vi "Global Fit Decays.vi"(6 "IRF":cluster{"t Array":dbl[], "IRF Array":dbl[]}, 8 "error in (no error)":errorcluster, 10 "Abort Fit":refnum<vi>, 11 "Decay Graph":refnum<vi>) -> (0 "Error Out":errorcluster, 1 "Reduced Chi^2":dbl, 2 "R^2":dbl, 3 "Best Fit Parameters":dbl[](array[numeric]), 4 "Fit Output Message":string, 5 "Aborted?":bool)   [LabVIEW 2021]
uses:
  AlliGator Settings List.ctl
  Fits/IRF(X)PSED/Decay Fit Options v2.ctl
  Fits/Decay Convolution/Decay Model.ctl
  Fits/Residual Type.ctl
  Fits/IRF(X)PSED/Fit Weights Type.ctl
  Fits/Non-linear Fitting Method v2.ctl
  Fits/Fit Calculation Method.ctl
  Fits/Non-linear Fitting Algorithm.ctl
  Fits/Global Fits/Global Fit Data.ctl
  Fits/Global Fits/Global Fit Parameters Information.ctl
  AlliGator Decay Fit Parameter Constraints 2.ctl
  Fits/IRF(X)PSED/Decay Fit Parameters In List.ctl
  AlliGator Variables List.ctl
  Graphs/XY Graph/XY Graph Add Multiplots with Names.vi
  Fits/Abort Fit Global.vi
  AlliGator Settings.lvlib
  Fits/Fits.lvlib
  AlliGator Decay Fit.lvlib
  Graphs/XY Graph/XY Graph Add-Ons.lvlib
  Time/Time.lvlib
  AlliGator Globals, Variables & Constants.lvlib
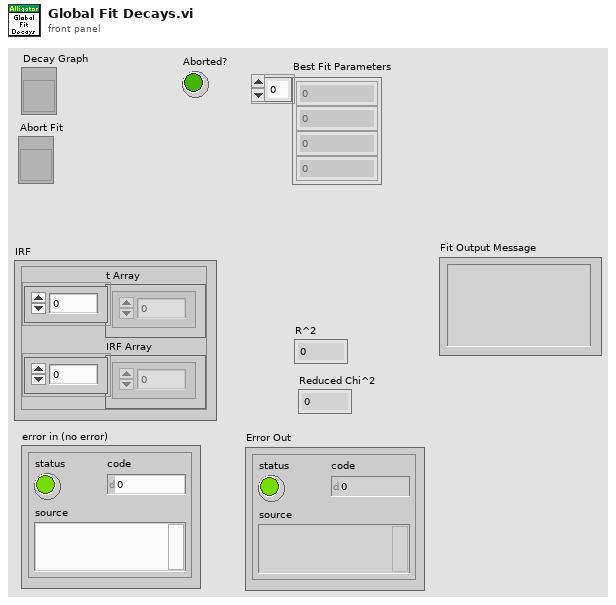
[diagram p1: front panel]
types:
  T1 = typedef "AlliGator Settings.lvlib/AlliGator Settings List.ctl" = enum16{"GUI:Visible Settings Tab", "GUI:Last Run Version", "Source Image:Use Image Histogram for Contrast", "Source Image:Low Count Pixels Rejection Options", "Source Image:High Count Pixels Rejection Options", "Source Image:Use Image Brightness", "Source Image:Blend Overlay with Image Background", "Source Image:Use Fixed ROI Diameter", "Source Image:ROI Diameter", "Source Image:ROI Center Color", "Source Image:Peak Threshold", "Source Image:Intensity Threshold", "Source Image:Image Binning Options", "Source Image:Image Smoothing Options", "Source Image:Image Histogram Active", "Source Image:Invert Binary Mask", "Source Image:Hot Pixel Removal", "Source Image:Overlay Analyzed ROI Center", "Source Image:Auto-Adjust Contrast", "Source Image:Histogram Lower Percentile", "Source Image:Histogram Upper Percentile", "Source Image:Save Source Image", "Source Image:Scale Bar Options", "Source Image:Image Resolution (Pixel Size)", "Source Image:Flatfield Correction", "Data Information:Gate Width", "Data Information:Nanotime Gate Separation", "Data Information:Macrotime Gate Separation", "Data Information:Gate Step", "Data Information:# Gates", "Data Information:Gate Image Exposure", "Data Information:Gate Image Integration", "Data Information:Gates to Skip", "Data Information:Gates to Keep", "Data Information:Define Gates to", "Data Information:Channel Name", "Data Information:Available Channel Names", "Data Information:Channel Arithmetic", "Data Information:Background File Subtraction", "Data Information:Background File", "Data Information:Background Scaling Factor", "Data Information:Background Pile-up Correction", "Data Information:Background Pixel Well Capacity", "Data Information:Laser Period", "Data Information:SYNC Period", "Data Information:Pile-up Correction", "Data Information:Pixel Well Capacity", "Data Information:Dataset Scaling Factor", "Fluorescence Decay_Decay Pre-Processing:Reverse Gates", "Fluorescence Decay_Decay Pre-Processing:Verbose Decay Pre-Processing", "Fluorescence Decay_Decay Pre-Processing:Use Decay Pre-Processing", "Fluorescence Decay_Decay Pre-Processing:Background Subtraction", "Fluorescence Decay_Decay Pre-Processing:Background Definition Range", "Fluorescence Decay_Decay Pre-Processing:Baseline Subtraction Method", "Fluorescence Decay_Decay Pre-Processing:Operations Order", "Fluorescence Decay_Decay Pre-Processing:Smoothing Parameter", "Fluorescence Decay_Decay Pre-Processing:Shift Decay", "Fluorescence Decay_Decay Pre-Processing:Decay Shift Parameters", "Fluorescence Decay_Decay Pre-Processing:Fold Decay", "Fluorescence Decay_Decay Pre-Processing:# Folds", "Fluorescence Decay_Decay Pre-Processing:1-Normalize Decay", "Fluorescence Decay_Decay Pre-Processing:[0-1]-Normalize Decay", "Fluorescence Decay_Decay Pre-Processing:Smoothen Decay", "Fluorescence Decay_Decay Pre-Processing:Extrapolate Decay", "Fluorescence Decay_Decay Pre-Processing:Use Periodicity", "Fluorescence Decay_Decay Pre-Processing:Use Cursors", "Fluorescence Decay_Decay Pre-Processing:Tail Fraction", "Fluorescence Decay_Decay Pre-Processing:Head Fraction", "Fluorescence Decay_Decay Pre-Processing:Additional Points", "Fluorescence Decay_Decay Pre-Processing:Straighten Decay", "Fluorescence Decay_Decay Pre-Processing:Constant Background", "Fluorescence Decay_Decay Pre-Processing:Pixel-Normalize Decay", "Fluorescence Decay_Advanced Analysis:Extract IRF instead of Decay", "Fluorescence Decay_Advanced Analysis:IRF Extraction Options", "Fluorescence Decay_Advanced Analysis:IRF Optimization Options", "Fluorescence Decay_Advanced Analysis:Square Pulse Options", "Fluorescence Decay_Advanced Analysis:IRF Order", "Fluorescence Decay_Advanced Analysis:IRF Time Constants", "Fluorescence Decay_Advanced Analysis:Wavelet Analysis Options", "Fluorescence Decay_Advanced Analysis:Average Lifetime Options", "Fluorescence Decay_Fit Options:Fit Options", "Fluorescence Decay_Fit Options:Use Legacy Fitting Approach", "Fluorescence Decay_Fit Options:Use Data Information Laser Period", "Fluorescence Decay_Fit Parameters:Displayed Fit Parameters", "Fluorescence Decay_Fit Parameters:Fit Parameter Constraints", "Fluorescence Decay_Fit Parameters:Export Tabulated Results", "Fluorescence Decay_Fit Parameters:MLE Baseline Offset Type", "Fluorescence Decay_Fit Parameters:MLE Baseline Offset", "Fluorescence Decay_Fit Parameters:Guess Parameter Names", "Fluorescence Decay_Fit Parameters:Guess Parameter Values", "Fluorescence Decay_Fit Parameters:Guess Parameters Options", "Fluorescence Decay_Styles:Show Last Decay Only", "Fluorescence Decay_Styles:Decay Graph Color Array", "Fluorescence Decay:Decay Graph Active", "Fluorescence Decay Statistics:Min Peak Value", "Fluorescence Decay Statistics:Reject Low Decay Peak Pixels", "Fluorescence Decay Statistics:Reject High Decay Peak Pixels", "Fluorescence Decay Statistics:Max Peak Value", "Time Traces:Use File Timestamp", "Time Traces:Time Step", "Time Traces:Use Intensity Correction File", "Time Traces:Intensity Correction File", "Phasor Plot:Phasor Plot Smoothing Options", "Phasor Plot:Phasor Plot Size", "Phasor Plot:Phasor Plot Graphics Options", "Phasor Plot:Cumulative Phasor Plot", "Phasor Plot:Use Phasor Brightness", "Phasor Plot:Blend Overlay with Phasor Background", "Phasor Plot:Save Phasor Plot", "Phasor Plot:Show References", "Phasor Plot:Phasor Ratio Decay Range", "Phasor Plot:Exponential Fading", "Phasor Plot:Phasor Ratio Reference Colors", "Phasor Plot:Reference Radius", "Phasor Plot:Show Color Map Vertices", "Phasor Plot:Phasor Plot Active", "Phasor Plot:Phasor Ratio Color Map Type", "Phasor Plot:Phasor Ratio Color Map", "Phasor Plot:Phasor Ratio Display Range", "Phasor Plot:Selected Image ROI(s)", "Phasor Plot:All Image ROIs", "Phasor Plot:Selected Phasor Plot ROI(s)", "Phasor Plot:All Phasor Plot ROIs", "Phasor Plot:Phasor Ratio Color-Coded Quantity", "Phasor Plot:Store Phasor Harmonics", "Phasor Plot:Draw Reference Segment", "Phasor Plot:User-Defined Quantity", "Phasor Graph:Phasor Frequency", "Phasor Graph:Phasor Ratio Type", "Phasor Graph:Pixel-level Phasor Computation", "Phasor Graph:Save Phasor Graph", "Phasor Graph:Phasor Graph Active", "Phasor Graph:Phasor SDV Options", "Phasor Calibration:Use Backup Calibration if needed", "Phasor Graph:Define Shortest Lifetime as", "Phasor Calibration:Backup Calibration Type", "Phasor Calibration:Calibration Type", "Phasor Calibration:Calibration Lifetime", "Phasor Calibration:Calibration Map Algorithm", "Single-Exponential Phasor Locus (SEPL):Gate Parameters", "Single-Exponential Phasor Locus (SEPL):User-defined Gate", "Single-Exponential Phasor Locus (SEPL):User-defined IRF", "Single-Exponential Phasor Locus (SEPL):Phasor Parameters", "Single-Exponential Phasor Locus (SEPL):Decay & IRF Parameters", "Single-Exponential Phasor Locus (SEPL):Display Parameters", "Lifetime Analysis:Decay Analysis Parameters", "Lifetime Analysis:Lifetime Map Active", "Plugins:Python Settings", "Miscellaneous:Verbose Mode", "Miscellaneous:Beep after Script", "Miscellaneous:Saved Image File Format", "Miscellaneous:Exported Gate Image Settings", "Miscellaneous:Include Loading in Timing", "Miscellaneous:Verbose Settings Mode", "Miscellaneous:Histogram Options", "Miscellaneous:Beep on Error", "Miscellaneous:# Logical Processors Used", "Miscellaneous:ROI Description Max Characters", "Miscellaneous:Verbose Error Mode", "Miscellaneous:Transparent Mask Color"}
  T2 = typedef "Fits.lvlib/Decay Fit Options v2.ctl" = cluster{"Show Fit Residuals":bool, "Fit Model":T3, "Residual Type":T4, "Max Decay Percentile":dbl, "Min Decay Percentile":dbl, "Show Full Decay":bool, "Weights":T5, "Fitting Method":T6, "Compute Parameter Uncertainties":bool, "Periodic Boundaries":bool, "Model Calculation":T7, "Period":dbl[unit], "Termination Criteria":cluster{"Max Iterations":i32, "Max Function Calls":i32, "Max Time":dbl[unit], "Function Tolerance":dbl, "Parameter Tolerance":dbl, "Gradient Tolerance":dbl, "Min Lambda":dbl, "Max Lambda":dbl, "Initial Tick Count":u32}, "Offset Resolution":dbl[unit], "Use Local IRF":bool, "Fitting Algorithm":T8}
  T3 = typedef "Fits.lvlib/Decay Model.ctl" = enum16{"1-Exponential", "2-Exponentials"}
  T4 = typedef "Fits.lvlib/Residual Type.ctl" = enum16{"Standard", "Normalized", "Reduced"}
  T5 = typedef "Fits.lvlib/Fit Weights Type.ctl" = enum16{"Unweighted", "1/Variance", "Best of All"}
  T6 = typedef "Fits.lvlib/Non-linear Fitting Method v2.ctl" = enum16{"Least Square", "Least Absolute Residual", "Bisquare", "MLE", "-", "Best of All"}
  T7 = typedef "Fits.lvlib/Fit Calculation Method.ctl" = enum16{"Simulation", "Convolution", "Integration"}
  T8 = typedef "Fits.lvlib/Non-linear Fitting Algorithm.ctl" = enum16{"Levenberg-Marquardt", "Trust-Region Dogleg"}
  T9 = cluster{"Max Iterations":i32, "Max Function Calls":i32, "Max Time":dbl[unit], "Function Tolerance":dbl, "Parameter Tolerance":dbl, "Gradient Tolerance":dbl, "Min Lambda":dbl, "Max Lambda":dbl, "Initial Tick Count":u32}
  T10 = typedef "XY Graph Add-Ons.lvlib/XY Graph Refnum.ctl" = refnum<vi>
  T11 = typedef "AlliGator Globals, Variables & Constants.lvlib/AlliGator Variables List.ctl" = enum16{"---- GUI ----", "Initialization Status", "State Indicators Refnum", "Original AlliGator Menu Items", "Current Action Loop State", "Script in progress", "Playback", "Loop Playback", "Search ROI Used", "Search ROI", "Decay Graph Max Legend Size", "Intensity Graph Max Legend Size", "Decay Statistics Graph Max Legend Size", "Phasor Graph Max Legend Size", "Phasor Ratio Graph Max Legend Size", "Lifetime Graph Max Legend Size", "---- Files ----", "Export Dataset Frames as Individual Files", "Show Batch Export Help Balloons", "Frames in Dataset", "ptu File Frame Start Indices", "Current Frame in Dataset", "Current Frame Timestamp", "------ Python Plugins ------", "Python Plugins Information", "Python Session", "Valid Python Session?", "---- Source Image ----", "Dataset Loaded", "Dataset Metadata", "Dataset Channel", "Dataset Data Description", "Background Dataset Metadata", "Background Dataset Channel", "Background Dataset Data Description", "Background File Subtraction", "Background File Path", "Background File Pile-up Correction", "Background File Pixel Well Capacity", "Background File Scaling Factor", "Source Image ROIs", "Current Source Image ROI", "Source Image ROI Event Refnum", "X_Source Image Display Range", "X_Source Image Palette Information", "Source Image Palette List", "Source Image Scale", "Current Dataset Load Settings", "Source Image:ROI Overlay Color", "---- Image Profile Window ----", "Image Profile:Overlay ROI in Source Image", "Image Profile Window Event Refnum", "Image Profile:IntensityType", "Image Profile:Intensity Average Type", "Image Profile:Intensity-weighted SDV", "Image Profile:Box Profile Type", "Image Profile Window Open", "Image Profile:Plotted Fit Parameter", "X_Type of Displayed Image", "X_Time Gate Slider", "Dataset Path", "Source Image Overlay to Erase", "Is Displayed Image Accumulated", "White Light Image Modified", "Mask Image Modified", "Macrotime Gate Separation", "------ Phasor Graph -------", "Phasor Graph:Show Line", "---- Phasor Plot ---", "Phasor Plot Parameters Changed", "FLI Dataset Modified since last Phasor Plot Calculation", "Phasor Harmonics Data", "Selected Phasor Harmonics", "Phasor Harmonic Manager Event Refnum", "Phasor Plot ROIs", "Current Phasor Plot ROI", "Phasor Plot ROI Event Refnum", "Phasor Plot Image Reference Points", "Phasor Plot Computed", "Phasor Plot Palette Information", "Phasor Plot Palette List", "Phasor Ratio Palette Information", "Phasor Ratio Palette List", "Phasor Image Scale", "Phasor Plot Image Overlay to Erase", "Phasor Plot Image Elements to Update", "Current Phasor Plot Calculation Parameters", "Current Phasor Calibration Options", "Reset Cumulated Phasor Plot", "Phasor Ratio Reference 1", "Phasor Ratio Lifetime Reference 1", "Phasor Ratio Reference 1 Frequency", "Phasor Ratio Reference 2", "Phasor Ratio Lifetime Reference 2", "Phasor Ratio Reference 2 Frequency", "---- Decay Analysis ----", "Number of Selected Decays to Fit", "LS Fit Results", "LAR Fit Results", "BS Fit Results", "Last Decay Max - Min", "Best Fit Parameters", "Best Fit Parameter Names", "Actual Size X", "Actual Size Y", "Binning X", "Binning Y", "Actual # Gates", "Dataset Number", "Gates to...", "Gates Skipped", "Gates to keep", "Gate Step", "Gate Separation", "Reversed Gates", "Pile-up Correction", "Pixel Well Capacity", "Background Subtracted", "Background Subtraction Method", "Background Definition Range", "Background File (deprecated)", "Number of Dataset Accumulated", "Array of Accumulated Dataset Paths", "Do Averaged Datasets", "Destination File Path", "Process Plot Target", "Use 1/D as Phasor Frequency", "---- Decay Fit Parameter Map -----", "Decay Fit Parameter Map Palette Information", "Decay Fit Parameter Map Palette List", "Local Decay Graph Window Event Refnum", "------- Local Decay Window ---------", "Use normalized IRF for convolution", "----- Miscellaneous ----", "Skippable Dialog Windows Status"}
  T12 = typedef "AlliGator Decay Analysis.lvlib/AlliGator Decay Fit.lvlib/AlliGator Decay Fit Parameter Constraints 2.ctl" = cluster{"Fit Parameter":T13, "Min Value":dbl, "Max Value":dbl, "Global":bool, "Used":bool}
  T13 = typedef "Fits.lvlib/Decay Fit Parameters In List.ctl" = enum16{"Offset", "Baseline", "A_1", "tau_1", "A_2", "tau_2"}
  T14 = typedef "Global Fit Data.ctl" = cluster{"Fit Data":variant, "Global Fit Parameter Information":T15, "# Points in Plots":i32[]}
  T15 = typedef "Fits.lvlib/Global Fit Parameters Information.ctl" = cluster{"Original Parameter Indices":i32[], "# Global Parameters":i32, "# Plot Specific Parameters":i32, "Global Parameter? Array":bool[]}
  T16 = cluster{"parameter minimum":dbl[], "parameter maximum":dbl[]}
  T17 = cluster{"t Array":dbl[], "Residual Array":dbl[]}[]
  T18 = typedef "Fits.lvlib/Non-linear Fit Output v3.ctl" = cluster{"best nonlinear fit":dbl[], "best fit parameters":dbl[], "R^2":dbl, "RMSE":dbl, "error out":errorcluster, "Fitting Method":T19, "number of function calls":i32, "number of iterations":i32, "covariance":T20, "Chi 2":dbl, "DOF":i32, "Fit Convergence Criterion":T21, "Fitting Algorithm":T8, "Weighted Fit":bool, "Gradient":dbl, "|Delta Chi 2|":dbl, "|Delta Chi 2|/Chi 2":dbl, "Max |Delta a| /|a|":dbl, "Lambda":dbl, "RSS":dbl, "AIC":dbl, "BIC":dbl, "Max number of function calls":i32, "Max number of iterations":i32, "IRF":T22, "IRF Normalization Factor":dbl, "Decay Normalization Factor":dbl}
  T19 = typedef "Fits.lvlib/Nonlinear Fit Method.ctl" = enum16{"Least Square", "Least Absolute Residual", "Bisquare", "MLE"}
  T20 = typedef "NI_Matrix.lvlib/RealMatrix.ctl" = dbl[][]
  T21 = typedef "Fits.lvlib/Convergence Criteria.ctl" = enum16{"Continue", "Tolerances Exceeded", "Max Time Exceeded", "Max Iterations Exceeded", "Max Function Evaluations Exceeded", "Scale Range Exceeded"}
  T22 = typedef "XY Graph Add-Ons.lvlib/XY Plot Data.ctl" = cluster{"X Array":dbl[], "Y Array":dbl[]}
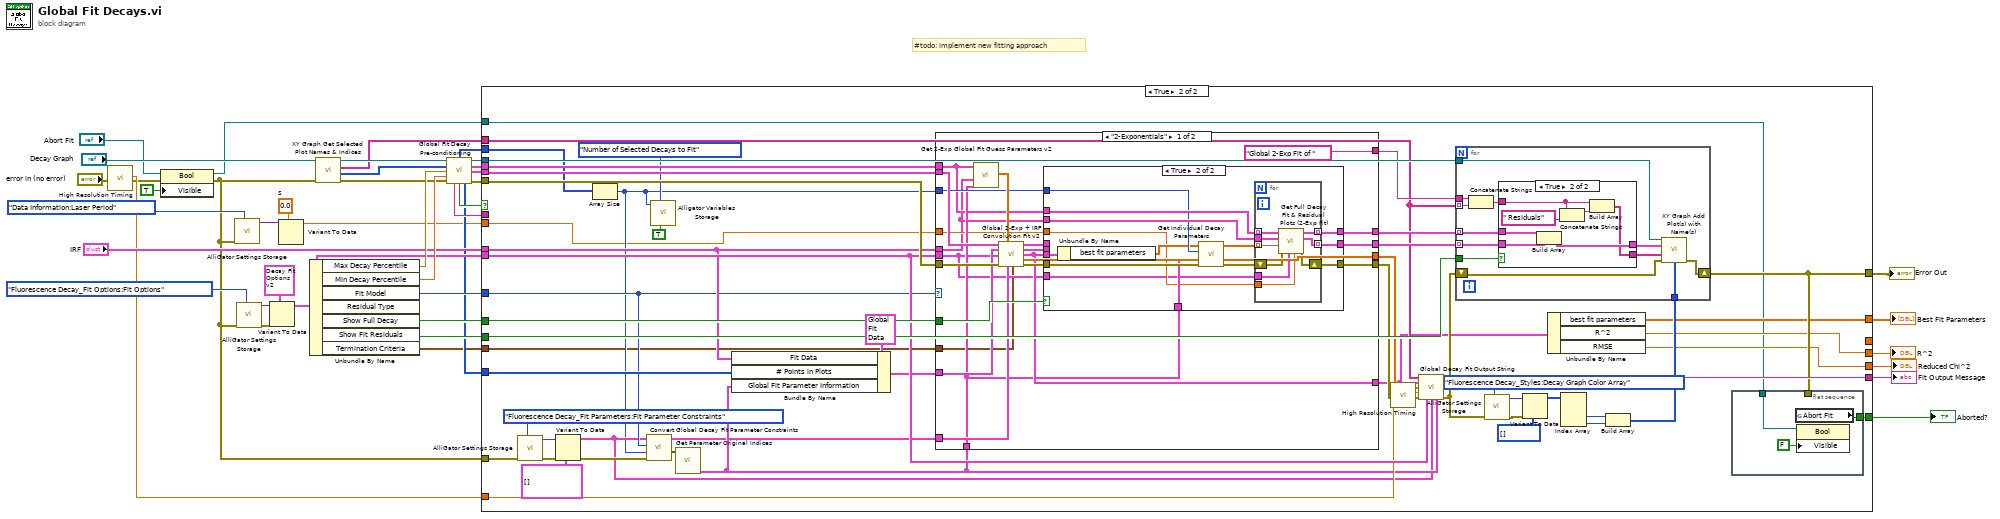
[diagram p0: block diagram]
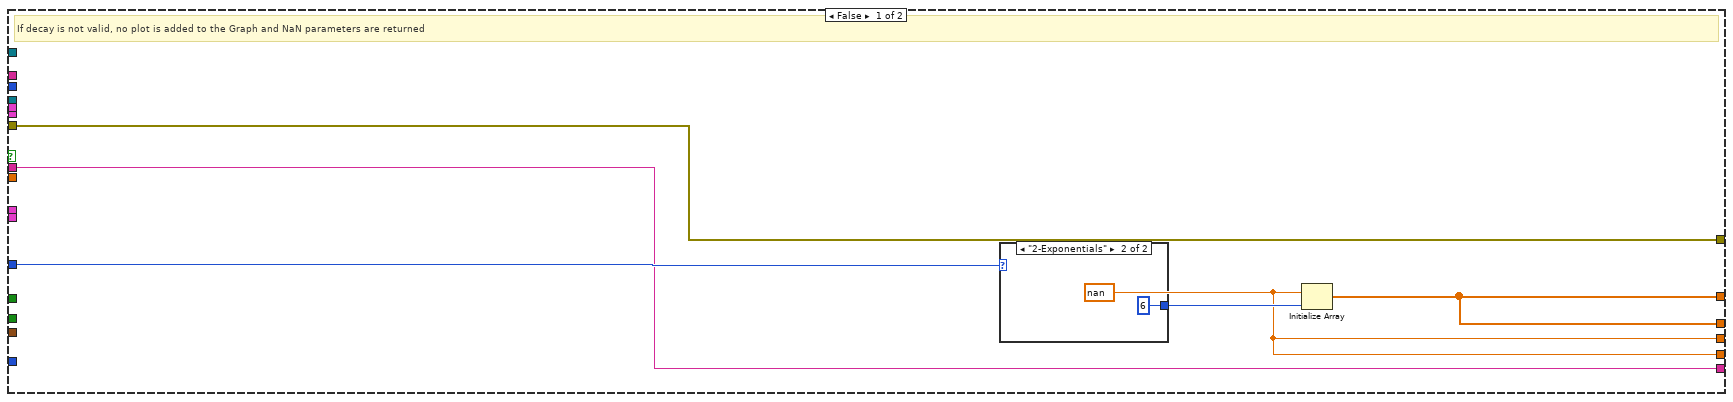
[diagram p2: hidden frame]
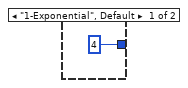
[diagram p3: hidden frame]
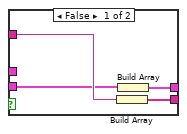
[diagram p4: hidden frame]
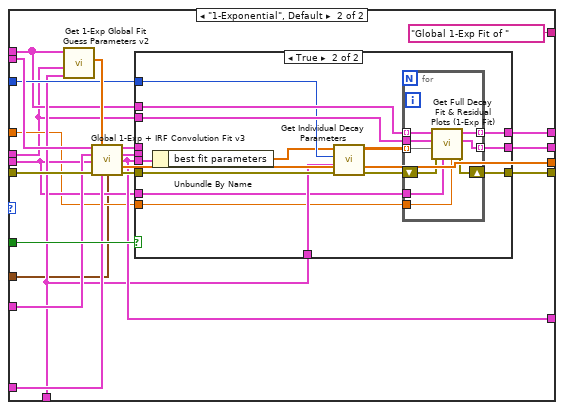
[diagram p6: hidden frame]
diagram:
  w8 = dbl[unit] 0.0  # s
  # "#todo: implement new fitting approach"
  n1 = call "High Resolution Timing.vi"("Error In"="error in (no error)") -> ("elapsed (relative) seconds"=w16:dbl, "Error Out"=w4:errorcluster)  [unwired: 16 in, 1 out]
  n2 = property class="Bool"(reference="Abort Fit", error in=w4, "Visible"=TRUE) -> (reference out=w2:refnum<vi>, error out=w3:errorcluster)
  n3 = call "AlliGator Settings Storage.vi"("AlliGator Settings List"=AlliGator_Settings_List."Data Information:Laser Period", "Error In"=w3) -> ("Variant Data out"=w9:variant)  [unwired: 8 in, 1 out]
  n4 = call "AlliGator Settings Storage.vi"("AlliGator Settings List"=AlliGator_Settings_List."Fluorescence Decay_Fit Options:Fit Options", "Error In"=w3) -> ("Error Out"=w37:errorcluster, "Variant Data out"=w38:variant)  [unwired: 8 in]
  n5 = Variant To Data(error in=w37, type=T2 {"Show Fit Residuals"=TRUE, "Fit Model"=enum."1-Exponential", "Residual Type"=enum."Standard", "Max Decay Percentile"=0.0, "Min Decay Percentile"=0.0, "Show Full Decay"=TRUE, "Weights"=enum."Unweighted", "Fitting Method"=enum."Least Square", "Compute Parameter Uncertainties"=TRUE, "Periodic Boundaries"=TRUE, "Model Calculation"=enum."Simulation", "Period"=1.2500000000000001e-08, "Termination Criteria"={"Max Iterations"=1000, "Max Function Calls"=0, "Max Time"=1000.0, "Function Tolerance"=1e-06, "Parameter Tolerance"=1e-06, "Gradient Tolerance"=0.0, "Min Lambda"=1e-06, "Max Lambda"=1e-06, "Initial Tick Count"=0}, "Offset Resolution"=1.2500000000000001e-08, "Use Local IRF"=TRUE, "Fitting Algorithm"=enum."Levenberg-Marquardt"} ("Fit Options"), Variant=w38) -> (data=w28:T2)  [unwired: 1 out]
  n6 = Variant To Data(type=w8, Variant=w9) -> (data=w7:dbl[unit])  [unwired: 1 in, 1 out]
  n7 = Unbundle By Name(w28) -> ("Max Decay Percentile"=w32:dbl, "Min Decay Percentile"=w31:dbl, "Fit Model"=w26:T3, "Show Full Decay"=w30:bool, "Show Fit Residuals"=w27:bool, "Termination Criteria"=w6:T9)  [unwired: 1 out]
  n8 = call "XY Graph Get Selected Plot Names & Indices.vi"("error in (no error)"=w3, "XYGraph in"="Decay Graph") -> ("error out"=w12:errorcluster, "Selected Plots"=w11:i32[], "Selected Plot Names"=w19:string[], "XYGraph out"=w24:T10)  [unwired: 5 in, 1 out]
  n9 = call "Global Fit Decay Pre-conditioning.vi"("XYGraph in"=w24, "Selected Plots"=w11, "Max Decay Percentile (1)"=w32, "Min Decay Percentile (0)"=w31, "error in (no error)"=w12) -> ("Index Max Array"=w20:i32[], "XYGraph out"=w42:refnum<vi>, "Full Decays"=w18:cluster{"t Array":dbl[], "Value Array":dbl[]}[], "Clipped Decays"=w22:cluster{"t Array":dbl[], "Value Array":dbl[]}[], "Message"=w23:string, "Is Valid?"=w29:bool, "# Points"=w13:i32[], "error out"=w14:errorcluster)  [unwired: 1 in, 2 out]
  n10 = case shown="True" w29 {
    tunnel: w42 -> [_ w103]
    tunnel: [w48 w85] -> w41
    tunnel: [w43 w100] -> w40
    tunnel: [w45 w56] -> w35
    tunnel: [w45 _] -> _
    tunnel: [w44 w55] -> w34
    tunnel: w26 -> [w47 w79]
    tunnel: [w44 w54] -> w33
    tunnel: "IRF" -> [_ w83]
    tunnel: w30 -> [_ w96]
    tunnel: w27 -> [_ w104]
    tunnel: w14 -> [w48 w95]
    tunnel: w28 -> [_ w93]
    tunnel: w23 -> [w43 _]
    tunnel: w22 -> [_ w92]
    tunnel: w20 -> [_ w59]
    tunnel: w19 -> [_ w90]
    tunnel: w18 -> [_ w91]
    tunnel: w16 -> [_ w88]
    tunnel: [_ w86] -> w15
    tunnel: w13 -> [_ w82]
    tunnel: w3 -> [_ w73]
    tunnel: w7 -> [_ w53]
    tunnel: w6 -> [_ w52]
    tunnel: w2 -> [_ w51]
    frame False {
      w44 = nan ("element")
      # "If decay is not valid, no plot is added to the Graph and NaN parameters are returned"
      n11 = case shown="\"2-Exponentials\"" w47 {
        tunnel: [4 ("dimension size") 6 ("dimension size")] -> w46
        frame "1-Exponential", Default {
        }
        frame "2-Exponentials" {
        }
      }
      n12 = Initialize Array(w44, w46) -> (w45:dbl[])
    }
    frame True {
      n13 = call "AlliGator Settings Storage.vi"("AlliGator Settings List"=AlliGator_Settings_List."Fluorescence Decay_Fit Parameters:Fit Parameter Constraints", "Error In"=w73) -> ("Error Out"=w75:errorcluster, "Variant Data out"=w76:variant)  [unwired: 8 in]
      n14 = Variant To Data(error in=w75, type=T12[] [] ("Fit Parameter Constraints"), Variant=w76) -> (data=w70:T12[], error out=w71:errorcluster)
      n15 = Array Size(array=w59) -> (size(s)=w58:i32)
      n16 = call "Convert Global Decay Fit Parameter Constraints.vi"("Error In"=w71, "# Plots"=w58, "Fit Model"=w79, "Fit Parameter Constraints"=w70) -> ("Global Parameters?"=w78:bool[], "Parameter Bounds"=w77:T16)  [unwired: 5 in, 1 out]
      n17 = call "Alligator Variables Storage.vi"("Get(F)/Set"=TRUE, "AlliGator Variable"=AlliGator_Variables_List."Number of Selected Decays to Fit" ("Alligator Variable"), "Data in"=w58) -> ()  [unwired: 6 in, 3 out]
      n18 = call "Get Parameter Original Indices.vi"("Parameter Types"=w78) -> ("Global Fit Parameter Info"=w80:T15)  [unwired: 8 in, 2 out]
      n19 = Bundle By Name(cluster=T14 {"Fit Data"=variant(cluster{"t Array":dbl[], "IRF Array":dbl[]} {"t Array"=[], "IRF Array"=[]}), "Global Fit Parameter Information"={"Original Parameter Indices"=[], "# Global Parameters"=0, "# Plot Specific Parameters"=0, "Global Parameter? Array"=[]}, "# Points in Plots"=[]} ("Global Fit Data"), "Fit Data"=w83, "# Points in Plots"=w82, "Global Fit Parameter Information"=w80) -> (w81:T14)
      n20 = case shown="\"2-Exponentials\"" w79 {
        tunnel: w83 -> [w131 w179]
        tunnel: w95 -> [w152 w200]
        tunnel: ["Global 2-Exp Fit of " ("string") "Global 1-Exp Fit of " ("string")] -> w102
        tunnel: [w146 w194] -> w101
        tunnel: [w145 w193] -> w94
        tunnel: [w150 w198] -> w98
        tunnel: [w147 w195] -> w99
        tunnel: w96 -> [w149 w197]
        tunnel: w93 -> [w134 w183]
        tunnel: w77 -> [w144 w192]
        tunnel: w92 -> [w141 w189]
        tunnel: w81 -> [w139 w187]
        tunnel: w80 -> [w136 w184]
        tunnel: w91 -> [w133 w181]
        tunnel: w58 -> [w138 w186]
        tunnel: [w137 w185] -> w57
        tunnel: w53 -> [w135 w182]
        tunnel: w52 -> [w132 w180]
        frame "2-Exponentials" {
          n21 = call "Get 2-Exp Global Fit Guess Parameters v2.vi"("Global Fit Parameter Info"=w136, "IRF"=w131, "Full Decays"=w133) -> ("Initial Parameters"=w140:dbl[])  [unwired: 8 in]
          n22 = call "Global 2-Exp + IRF Convolution Fit v2.vi"("Decays"=w141, "Initial Parameters"=w140, "Global Fit Parameters Info"=w139, "Fit Options"=w134, "error in (no error)"=w152, "parameter bounds"=w144, "Termination Criteria"=w132) -> ("Fitted Decays"=w143:cluster{"t Array":dbl[], "Fitted Array":dbl[]}[], "Residuals"=w148:T17, "Fit Output"=w137:T18, "Delta Best Fit Parameters"=w150:dbl[], "error out"=w142:errorcluster)  [unwired: 4 in]
          n23 = case shown="True" w149 {
            tunnel: w143 -> [w154 _]
            tunnel: w148 -> [w153 _]
            tunnel: [w154 w162] -> w147
            tunnel: [w153 w161] -> w146
            tunnel: w142 -> [w155 w167]
            tunnel: [w155 w169] -> w145
            tunnel: w131 -> [_ w168]
            tunnel: w136 -> [_ w166]
            tunnel: w133 -> [_ w164]
            tunnel: w138 -> [_ w160]
            tunnel: w137 -> [_ w159]
            tunnel: w135 -> [_ w157]
            tunnel: w134 -> [_ w156]
            frame False {
            }
            frame True {
              n24 = Unbundle By Name(w159) -> ("best fit parameters"=w158:dbl[])
              n25 = call "Get Individual Decay Parameters.vi"("Error In"=w167, "Global Fit Parameter Info"=w166, "# Decays"=w160, "Global Fit Parameters Array"=w158) -> ("Error Out"=w163:errorcluster, "All Parameters Array"=w165:dbl[][])  [unwired: 4 in, 2 out]
              n26 = for {
                tunnel: w168 -> [w178]
                tunnel: w165 -> [w177] mode=indexing
                tunnel: w164 -> [w176] mode=indexing
                shift-right: [w174] -> w169
                shift-left: w163 -> [w175]
                tunnel: [w173] -> w162 mode=indexing
                tunnel: [w172] -> w161 mode=indexing
                tunnel: w157 -> [w171]
                tunnel: w156 -> [w170]
                n27 = call "Get Full Decay Fit & Residual Plots (2-Exp Fit).vi"("Laser Period"=w171, "Fit Options"=w170, "Error In"=w175, "Best Fit Parameters"=w177, "IRF"=w178, "Full Decay"=w176) -> ("Error Out"=w174:errorcluster, "Full Decay Residuals"=w172:cluster{"t Array":dbl[], "IRF Array":dbl[]}, "Full Fitted Decay"=w173:cluster{"t Array":dbl[], "IRF Array":dbl[]})  [unwired: 3 in]
              }
            }
          }
        }
        frame "1-Exponential", Default {
          n28 = call "Get 1-Exp Global Fit Guess Parameters v2.vi"("Global Fit Parameter Info"=w184, "IRF"=w179, "Full Decays"=w181) -> ("Initial Parameters"=w188:dbl[])  [unwired: 8 in]
          n29 = call "Global 1-Exp + IRF Convolution Fit v3.vi"("Decays"=w189, "Initial Parameters"=w188, "Global Fit Parameters Info"=w187, "Fit Options"=w183, "error in (no error)"=w200, "parameter bounds"=w192, "Termination Criteria"=w180) -> ("Fitted Decays"=w191:cluster{"t Array":dbl[], "Fitted Array":dbl[]}[], "Residuals"=w196:T17, "Fit Output"=w185:T18, "Delta Best Fit Parameters"=w198:dbl[], "error out"=w190:errorcluster)  [unwired: 4 in]
          n30 = case shown="True" w197 {
            tunnel: w191 -> [w202 _]
            tunnel: w196 -> [w201 _]
            tunnel: [w202 w210] -> w195
            tunnel: [w201 w209] -> w194
            tunnel: w190 -> [w203 w215]
            tunnel: [w203 w217] -> w193
            tunnel: w179 -> [_ w216]
            tunnel: w184 -> [_ w214]
            tunnel: w181 -> [_ w212]
            tunnel: w186 -> [_ w208]
            tunnel: w185 -> [_ w207]
            tunnel: w183 -> [_ w205]
            tunnel: w182 -> [_ w204]
            frame False {
            }
            frame True {
              n31 = Unbundle By Name(w207) -> ("best fit parameters"=w206:dbl[])
              n32 = call "Get Individual Decay Parameters.vi"("Error In"=w215, "Global Fit Parameter Info"=w214, "# Decays"=w208, "Global Fit Parameters Array"=w206) -> ("Error Out"=w211:errorcluster, "All Parameters Array"=w213:dbl[][])  [unwired: 4 in, 2 out]
              n33 = for {
                tunnel: w216 -> [w226]
                tunnel: w213 -> [w225] mode=indexing
                tunnel: w212 -> [w224] mode=indexing
                shift-right: [w222] -> w217
                shift-left: w211 -> [w223]
                tunnel: [w221] -> w210 mode=indexing
                tunnel: [w220] -> w209 mode=indexing
                tunnel: w205 -> [w219]
                tunnel: w204 -> [w218]
                n34 = call "Get Full Decay Fit & Residual Plots (1-Exp Fit).vi"("Laser Period"=w218, "Fit Options"=w219, "Error In"=w223, "Best Fit Parameters (All)"=w225, "IRF"=w226, "Full Decay"=w224) -> ("Error Out"=w222:errorcluster, "Full Decay Residuals"=w220:cluster{"t Array":dbl[], "Y Array":dbl[]}, "Full Fitted Decay"=w221:cluster{"t Array":dbl[], "Y Array":dbl[]})  [unwired: 3 in]
              }
            }
          }
        }
      }
      n35 = call "High Resolution Timing.vi"("relative seconds (NaN)"=w88, "Error In"=w94) -> ("elapsed (relative) seconds"=w87:dbl, "Error Out"=w89:errorcluster)  [unwired: 15 in, 1 out]
      n36 = call "Global Decay Fit Output String.vi"("Plot Names"=w90, "Fit Output"=w57, "Delta Best Fit Parameters"=w98, "elapsed (relative) seconds"=w87, "Error In"=w89, "Fit Options"=w93, "Fit Parameter Constraints"=w70, "Global Fit Parameter Info"=w80) -> ("Fit Output Message"=w100:string, "Error Out"=w62:errorcluster)  [unwired: 6 in]
      n37 = call "AlliGator Settings Storage.vi"("AlliGator Settings List"=AlliGator_Settings_List."Fluorescence Decay_Styles:Decay Graph Color Array", "Error In"=w62) -> ("Error Out"=w68:errorcluster, "Variant Data out"=w67:variant)  [unwired: 8 in]
      n38 = Variant To Data(error in=w68, type=u32[] [] ("appended array"), Variant=w67) -> (data=w69:u32[])  [unwired: 1 out]
      n39 = Unbundle By Name(w57) -> ("best fit parameters"=w56:dbl[], "R^2"=w55:dbl, "RMSE"=w54:dbl)
      n40 = Index Array(array=w69) -> (element #2=w64:u32, element #3=w63:u32)  [unwired: 3 in, 1 out]
      n41 = Build Array(w64, w63) -> (w97:u32[])
      n42 = for {
        tunnel: w104 -> [w119]
        tunnel: w103 -> [w113]
        tunnel: w102 -> [w118]
        tunnel: w101 -> [w117] mode=indexing
        tunnel: w99 -> [w116] mode=indexing
        tunnel: w97 -> [w110]
        shift-right: [w111] -> w85
        shift-left: w62 -> [w112]
        tunnel: w90 -> [w114] mode=indexing
        n43 = Concatenate Strings(w118, w114) -> (w115:string)
        n44 = case shown="True" w119 {
          tunnel: w117 -> [w121 w124]
          tunnel: [w120 w130] -> w109
          tunnel: w116 -> [_ w125]
          tunnel: w115 -> [w123 w128]
          tunnel: [w122 w126] -> w108
          frame False {
            n45 = Build Array(w123) -> (w122:string[])
            n46 = Build Array(w121) -> (w120:cluster{"t Array":dbl[], "Y Array":dbl[]}[])
          }
          frame True {
            n47 = Build Array(w125, w124) -> (w130:cluster{"t Array":dbl[], "Y Array":dbl[]}[])
            n48 = Concatenate Strings(w128, " Residuals" ("string")) -> (w127:string)
            n49 = Build Array(w128, w127) -> (w126:string[])
          }
        }
        n50 = call-poly "XY Graph Add Plot(s) with Name(s).vi"("XYGraph in"=w113, "Array of Plots"=w109, "Array of Plot Names (\"Plot\")"=w108, "error in (no error)"=w112, "Plot Colors (Default)"=w110) -> ("error out"=w111:errorcluster)  [unwired: 6 in, 4 out]
      }
      n51 = flat-sequence {
        tunnel: [w107] -> w86
        tunnel: w85 -> [_]
        tunnel: w51 -> [w105]
        frame #0 {
          n52 = global read "Abort Fit Global.vi" "Abort Fit"() -> (w107:bool)
          n53 = property class="Bool"(reference=w105, "Visible"=FALSE) -> ()  [unwired: 1 in, 2 out]
        }
      }
    }
  }
  "Error Out" <- w41
  "Fit Output Message" <- w40
  "Best Fit Parameters" <- w35
  "R^2" <- w34
  "Reduced Chi^2" <- w33
  "Aborted?" <- w15
